vi "File.Copy Source to Dest, Changed Files Only.vi"(8 "error in":errorcluster, 9 "Type":enum16{"Merge", "Match"}(ring), 10 "Dest Folder":path, 11 "Source Folder":path) -> (0 "error out":errorcluster, 1 "Report":string, 2 "Copied Files":path[](array[path]), 3 "Copy Count":i32, 4 "Deleted Files":path[](array[path]), 5 "Delete Count":i32)   [LabVIEW 2024, in "KATE_Lib.lvlib" / "File Utils.lvlib"]
uses:
  File Utils.lvlib
  Status/Status Utils.lvlib
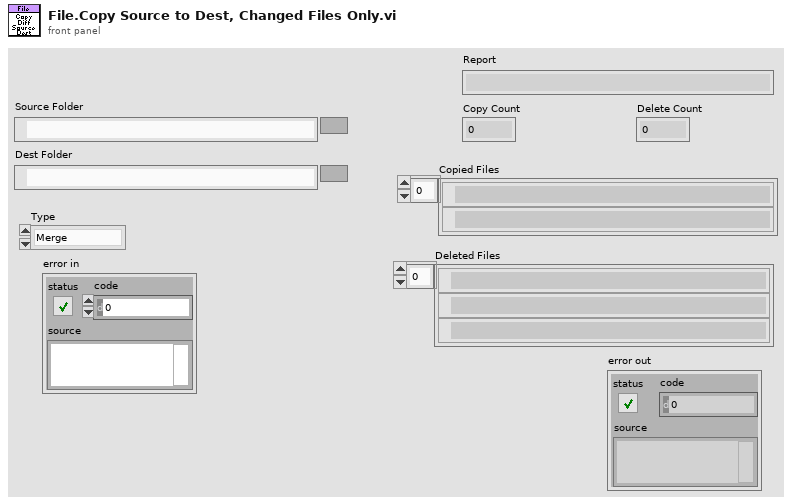
[diagram p1: front panel]
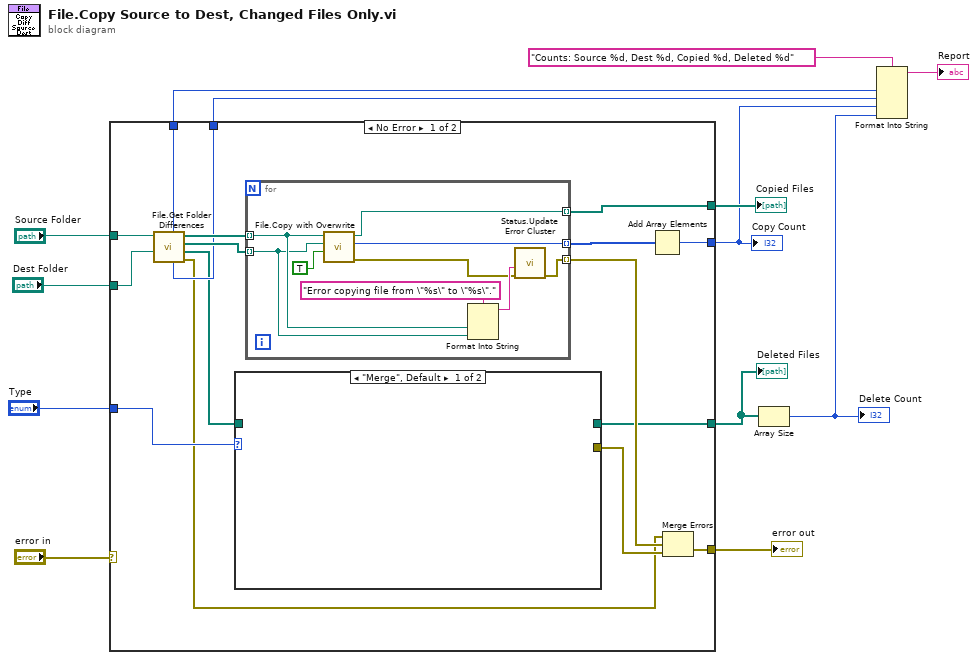
[diagram p0: block diagram]
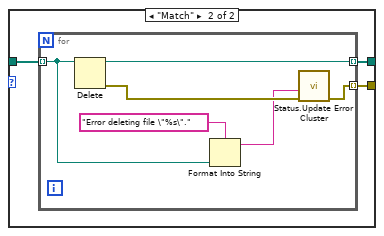
[diagram p2: hidden frame]
diagram:
  n1 = case shown="No Error" "error in" {
    selector: "error in" -> [_ w48]
    tunnel: "Source Folder" -> [w29 _]
    tunnel: "Dest Folder" -> [w28 _]
    tunnel: [w25 _] -> w3
    tunnel: [w24 w48] -> w10
    tunnel: [w23 _] -> w9
    tunnel: "Type" -> [w19 _]
    tunnel: [w18 _] -> w7
    tunnel: [w17 _] -> w5
    tunnel: [w16 _] -> w4
    frame No Error {
      n2 = call "File.Get Folder Differences.vi"("Dest Folder"=w28, "Source Folder"=w29) -> ("error out"=w14:errorcluster, "Dest not in Source"=w15:path[], "Dest"=w21:path[], "Source"=w22:path[], "Dest Cnt"=w16:i32, "Source Cnt"=w17:i32)  [unwired: 4 in]
      n3 = case shown="\"Merge\", Default" w19 {
        tunnel: w15 -> [_ w32]
        tunnel: [_ w31] -> w20
        tunnel: [_ w30] -> w18
        frame "Merge", Default {
        }
        frame "Match" {
          n4 = for {
            tunnel: w32 -> [w34] mode=indexing
            tunnel: [w37] -> w31 mode=indexing
            tunnel: [w38] -> w30 mode=indexing
            n5 = Delete(path (use dialog)=w34) -> (deleted path=w38:path, error out=w36:errorcluster)  [unwired: 4 in, 1 out]
            n6 = Format Into String(format string="Error deleting file \"%s\".", w34) -> (resulting string=w33:string)  [unwired: 2 in, 1 out]
            n7 = call "Status.Update Error Cluster.vi"("Error In"=w36, "NewDesc"=w33) -> ("Error Out"=w37:errorcluster)  [unwired: 9 in]
          }
        }
      }
      n8 = for {
        tunnel: w22 -> [w42] mode=indexing
        tunnel: w21 -> [w39] mode=indexing
        tunnel: [w46] -> w27 mode=indexing
        tunnel: [w41] -> w26 mode=indexing
        tunnel: [w45] -> w23 mode=indexing
        n9 = call "File.Copy with Overwrite.vi"("Dest is Dir(F)/File(T)"=TRUE, "Destination"=w39, "Source"=w42) -> ("error out"=w40:errorcluster, "Files Copied"=w46:i32, "Destination Dup"=w45:path)  [unwired: 6 in]
        n10 = Format Into String(format string="Error copying file from \"%s\" to \"%s\".", w42, w39) -> (resulting string=w43:string)  [unwired: 2 in, 1 out]
        n11 = call "Status.Update Error Cluster.vi"("Error In"=w40, "NewDesc"=w43) -> ("Error Out"=w41:errorcluster)  [unwired: 9 in]
      }
      n12 = Add Array Elements(numeric array=w27) -> (sum=w25:i32)
      n13 = Merge Errors(w14, w26, w20) -> (w24:errorcluster)
    }
    frame Error {
    }
  }
  "Copy Count" <- w3
  "error out" <- w10
  "Copied Files" <- w9
  "Deleted Files" <- w7
  n14 = Array Size(array=w7) -> (size(s)=w2:i32)
  "Delete Count" <- w2
  n15 = Format Into String(format string="Counts: Source %d, Dest %d, Copied %d, Deleted %d", w5, w4, w3, w2) -> (resulting string=→"Report":string)  [unwired: 2 in, 1 out]
